vi "readFromXML.vi"(8 "error in (no error)":errorcluster, 10 "XML in":string="<Planet>\n  <planetName>Venus</planetName>\n</Planet>", 11 "Planet in":refnum<class "Planet.lvclass">) -> (0 "error out":errorcluster, 3 "Planet out":refnum<class "Planet.lvclass">)   [LabVIEW 2022 SP3, in "TCSDataDefinitions.lvlib" / "TCSCommand.lvlib" / "TargetConfiguration.lvlib" / "Target.lvlib" / "Planet.lvclass"]
uses:
  Planet.lvclass
  Enumerations/PlanetNameValues.ctl
  Planet.lvclass/Planet.ctl
  Target/Target.lvclass
  <userlib>/Common/XML/XMLParser/XMLParser.lvclass
  Target.lvlib
panel:
  out "planetName":T1
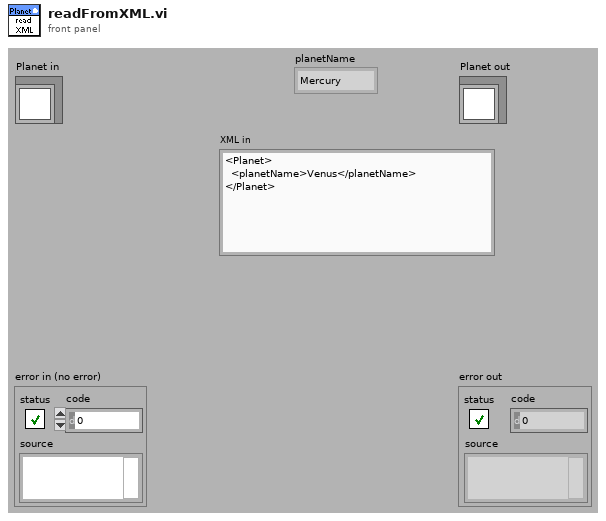
[diagram p1: front panel]
types:
  T1 = typedef "TCSDataDefinitions.lvlib/TCSCommand.lvlib/TargetConfiguration.lvlib/Target.lvlib/PlanetNameValues.ctl" = enum16{"Mercury", "Venus", "Moon", "Mars", "Jupiter", "Saturn", "Uranus", "Neptune", "Pluto"}
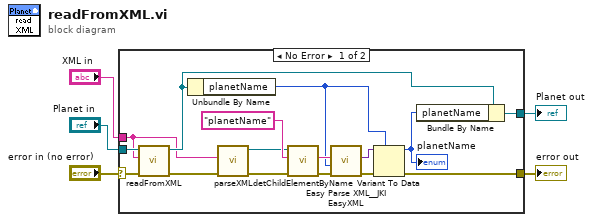
[diagram p0: block diagram]
diagram:
  n1 = case shown="No Error" "error in (no error)" {
    selector: "error in (no error)" -> [w15 w23]
    tunnel: [w12 w23] -> w4
    tunnel: [w19 w22] -> w2
    tunnel: "Planet in" -> [w18 w22]
    tunnel: "XML in" -> [w16 _]
    frame No Error {
      n2 = call-parent "readFromXML.vi"("error in (no error)"=w15, "XML in"=w16, "Target in"=w18) -> ("error out"=w14:errorcluster, "Target out"=w17:refnum<class "Planet.lvclass">)  [unwired: 7 out]
      n3 = Unbundle By Name(w17) -> ("planetName"=w9:T1)
      n4 = call <userlib>:"parseXML.vi"("error in (no error)"=w14, "XMLString in"=w16) -> ("error out"=w20:errorcluster, "Element out"=w6:refnum<class "XMLParser.lvclass">)  [unwired: 8 in]
      n5 = call <userlib>:"detChildElementByName.vi"("error in (no error)"=w20, "childName"="planetName" ("ChildName"), "Element in"=w6) -> ("error out"=w10:errorcluster, "childXML"=w11:string)  [unwired: 5 in, 2 out]
      n6 = call <vilib>:"Easy Parse XML__JKI EasyXML.vi"("error in (no error)"=w10, "LabVIEW Data (Type)"=w9, "XML String"=w11) -> ("error out"=w7:errorcluster, "LabVIEW Data"=w8:variant)  [unwired: 7 in]
      n7 = Variant To Data(error in=w7, type=w9, Variant=w8) -> (data=w13:T1, error out=w12:errorcluster)
      "planetName" <- w13
      n8 = Bundle By Name(cluster=w17, "planetName"=w13) -> (w19:refnum<class "Planet.lvclass">)
    }
    frame Error {
    }
  }
  "error out" <- w4
  "Planet out" <- w2
